vi "Init.vi"(8 "error in (no error)":errorcluster, 9 "SA Pin":string, 10 "Measurement Name":string) -> (0 "error out":errorcluster, 3 "GSM_ORFS_Custom out":refnum<class "GSM_ORFS_Custom.lvclass">)   [LabVIEW 2016, in "SeqAuto Evaluations.lvlib" / "GSM_ORFS_Custom.lvclass"]
uses:
  GSM_ORFS_Custom.lvclass
  C:/Sequence Automation/Plugins/SeqAuto IEvaluation.lvlibp/SeqAuto IEvaluation.lvclass
  GSM_ORFS_Custom.lvclass/GSM_ORFS_Custom.ctl
  Plugins/SeqAuto IEvaluation.lvlibp/Write Measurement Name.vi
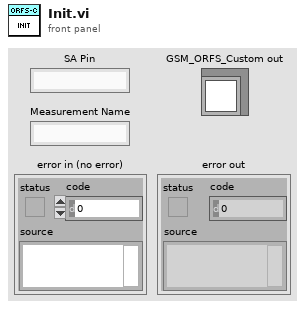
[diagram p1: front panel]
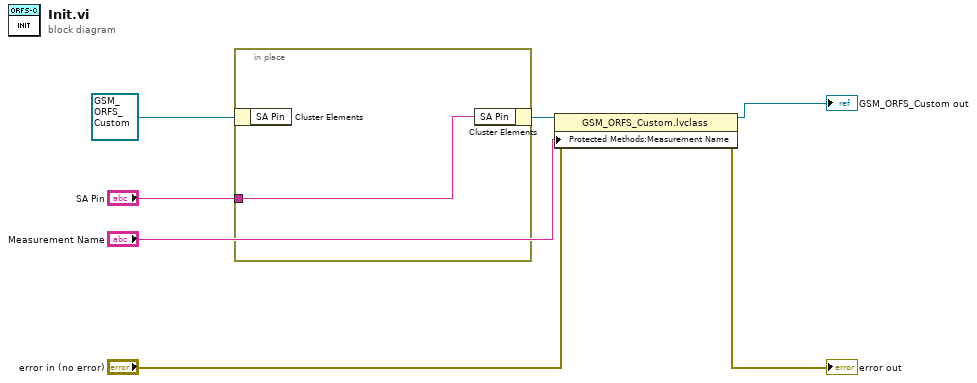
[diagram p0: block diagram]
diagram:
  n1 = in-place {
    in-place-border: "SA Pin" -> [w8]
    n2 = in-place-cluster #1(refnum<class "GSM_ORFS_Custom.lvclass"> refnum ("GSM_ORFS_Custom in")) -> ()  [unwired: 1 out]
    n3 = in-place-cluster #1("SA Pin"=w8) -> (w3:refnum<class "GSM_ORFS_Custom.lvclass">)
  }
  n4 = property class="GSM_ORFS_Custom.lvclass"(reference=w3, error in="error in (no error)", "Protected Methods:Measurement Name"="Measurement Name") -> (reference out=→"GSM_ORFS_Custom out":refnum<class "GSM_ORFS_Custom.lvclass">, error out=→"error out":errorcluster)
